vi "GetPersonAvgTime.vi"(7 "TimeToCheck":enum16{"AckTime", "FulfilledTime"}(ring)=enum."FulfilledTime", 8 "error in":errorcluster, 9 "To":timestamp, 10 "From":timestamp, 11 "PersonnelName":string) -> (0 "error out":errorcluster, 1 "NumOfRequests":i32, 2 "AvgTime(s)":dbl, 4 "NumOfAlarms":i32)   [LabVIEW 2015, in "DatabaseApi.lvlib"]
uses:
  DatabaseApi.lvlib
  TypeDef/Request/RequestsFilter.ctl
  TypeDef/Request/RequestsTableColumnNamesRing.ctl
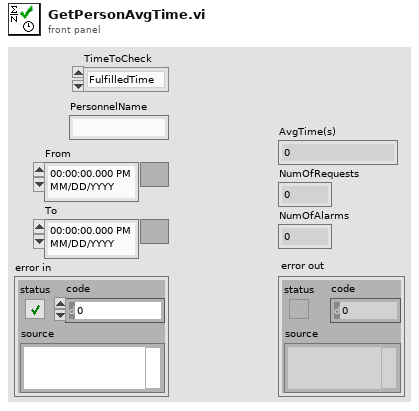
[diagram p1: front panel]
types:
  T1 = typedef "DatabaseApi.lvlib/RequestsTableColumnNamesRing.ctl" = enum16{"RequestID", "PersonnelType", "StartTime", "StartName", "AckTime", "AckName", "FulfilledTime", "FulfilledName", "Description", "Room Number", "Request Type", "Alarm"}
  T2 = typedef "DatabaseApi.lvlib/RequestsFilter.ctl" = cluster{"Filter":T1, "From":timestamp, "To":timestamp, "Filter Text":string, "Enable Filter":bool}
  T3 = typedef "Request.lvclass/RequestCluster.ctl" = cluster{"RequestID":string, "PersonelType":T4, "StartTime":timestamp, "StartName":string, "AckTime":timestamp, "AckName":string, "FulfilledTime":timestamp, "FulfilledName":string, "Description":string, "Room Number":i32, "Request Type":T5, "Alarm":bool}
  T4 = typedef "Request.lvclass/PersonnelType.ctl" = u16
  T5 = typedef "Request.lvclass/RequestType.ctl" = enum16{"Specific Call To Room", "General Call To Room"}
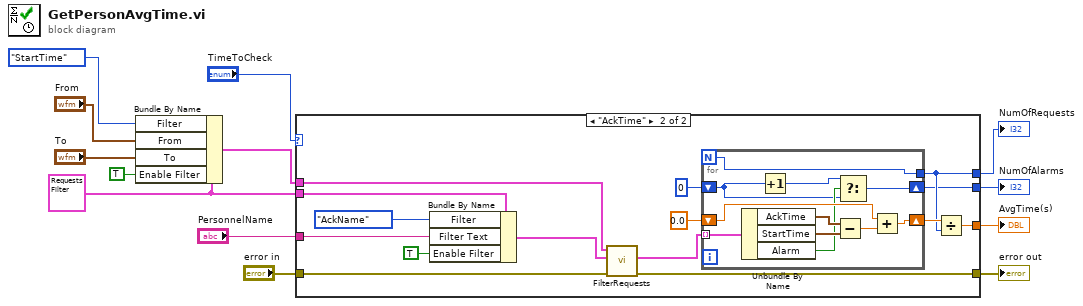
[diagram p0: block diagram]
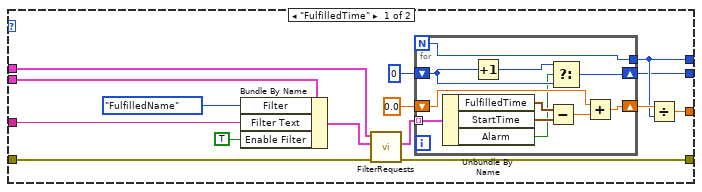
[diagram p2: hidden frame]
diagram:
  w8 = T2 {"Filter"=enum."StartTime", "From"=timestamp(0 s since 1904-01-01), "To"=timestamp(0 s since 1904-01-01), "Filter Text"="", "Enable Filter"=FALSE} ("Filter 3")
  n1 = Bundle By Name(cluster=w8, "Filter"=RequestsTableColumnNamesRing."StartTime", "From"="From", "To"="To", "Enable Filter"=TRUE) -> (w11:T2)
  n2 = case shown="\"AckTime\"" "TimeToCheck" {
    tunnel: "error in" -> [w28 w54]
    tunnel: [w27 w53] -> w12
    tunnel: w11 -> [w26 w52]
    tunnel: w8 -> [w25 w51]
    tunnel: "PersonnelName" -> [w22 w48]
    tunnel: [w17 w43] -> w6
    tunnel: [w16 w42] -> w2
    tunnel: [w14 w40] -> w1
    frame "FulfilledTime" {
      n3 = Bundle By Name(cluster=w25, "Filter"=RequestsTableColumnNamesRing."FulfilledName", "Filter Text"=w22, "Enable Filter"=TRUE) -> (w23:T2)
      n4 = call "FilterRequests.vi"("error in"=w28, "Filter 2"=w23, "Filter 1"=w26) -> ("error out"=w27:errorcluster, "Requests"=w20:T3[])  [unwired: 7 in]
      n5 = for {
        N -> [w34]
        tunnel: w20 -> [w39] mode=indexing
        shift-right: [w33] -> w18
        shift-left: 0.0 -> [w35]
        tunnel: [w34] -> w16
        shift-right: [w32] -> w14
        shift-left: 0 -> [w30]
        n6 = Unbundle By Name(w39) -> ("FulfilledTime"=w38:timestamp, "StartTime"=w37:timestamp, "Alarm"=w29:bool)
        n7 = Increment(x=w30) -> (x+1=w31:i32)
        n8 = Subtract(x=w38, y=w37) -> (x-y=w36:dbl)
        n9 = Select(t=w31, s=w29, f=w30) -> (s? t:f=w32:i32)
        n10 = Add(x=w35, y=w36) -> (x+y=w33:dbl)
      }
      n11 = Divide(x=w18, y=w16) -> (x/y=w17:dbl)
    }
    frame "AckTime" {
      n12 = Bundle By Name(cluster=w51, "Filter"=RequestsTableColumnNamesRing."AckName", "Filter Text"=w48, "Enable Filter"=TRUE) -> (w49:T2)
      n13 = call "FilterRequests.vi"("error in"=w54, "Filter 2"=w49, "Filter 1"=w52) -> ("error out"=w53:errorcluster, "Requests"=w46:T3[])  [unwired: 7 in]
      n14 = for {
        N -> [w60]
        tunnel: w46 -> [w65] mode=indexing
        shift-right: [w59] -> w44
        shift-left: 0.0 -> [w61]
        tunnel: [w60] -> w42
        shift-right: [w57] -> w40
        shift-left: 0 -> [w56]
        n15 = Unbundle By Name(w65) -> ("AckTime"=w64:timestamp, "StartTime"=w63:timestamp, "Alarm"=w58:bool)
        n16 = Increment(x=w56) -> (x+1=w55:i32)
        n17 = Subtract(x=w64, y=w63) -> (x-y=w62:dbl)
        n18 = Select(t=w55, s=w58, f=w56) -> (s? t:f=w57:i32)
        n19 = Add(x=w61, y=w62) -> (x+y=w59:dbl)
      }
      n20 = Divide(x=w44, y=w42) -> (x/y=w43:dbl)
    }
  }
  "error out" <- w12
  "AvgTime(s)" <- w6
  "NumOfRequests" <- w2
  "NumOfAlarms" <- w1
